vi "Write Data.vi"(8 "error in (no error)":errorcluster, 9 "Publication Time":timestamp, 10 "Value":variant, 11 "TerminalReference in":refnum<class "NamedNumericStringsBinding.lvclass">) -> (0 "error out":errorcluster, 3 "TerminalReference out":refnum<class "NamedNumericStringsBinding.lvclass">)   [LabVIEW 2017, in "Transport.lvlib" / "NamedNumericStringsBinding.lvclass"]
doc: "<License>\nCopyright © 2017 Composed Systems, LLC | All rights reserved\nwww.composed.io\n\nAuthor: Ethan Stern <ethan.stern@composed.io>\n\nThis software is provided \"AS IS\" WITHOUT WARRANTIES, either express or implied, AND IS FOR EDUCATIONAL PURPOSES ONLY.\n</License>MVA Framework 1.0.4.16\nEthan Stern - Composed Systems\nCopyright (c) 2017, Composed Systems"
uses:
  NamedNumericStringsBinding.lvclass
  NamedNumericStringsBinding.lvclass/NamedNumericStringsBinding.ctl
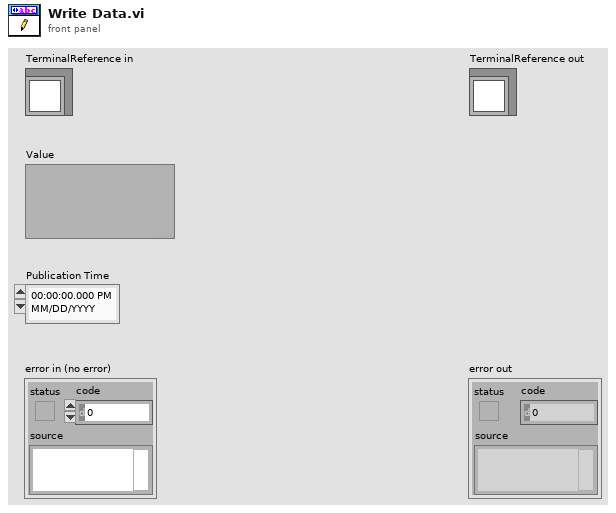
[diagram p1: front panel]
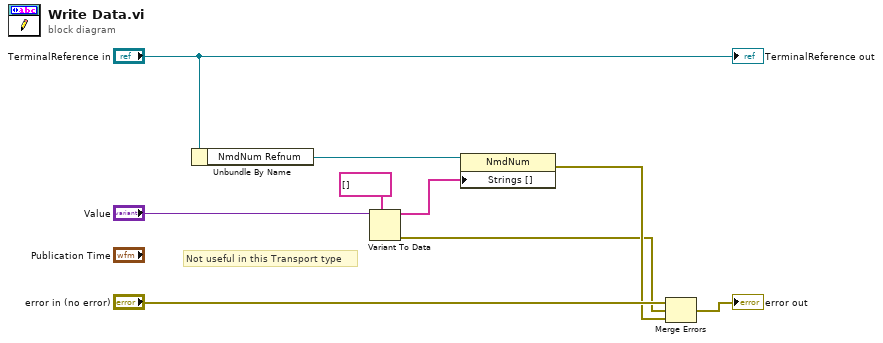
[diagram p0: block diagram]
diagram:
  # "Not useful in this Transport type"
  n1 = Unbundle By Name("TerminalReference in") -> ("NmdNum Refnum"=w7:refnum<vi>)
  n2 = Variant To Data(type=string[] [] ("Strings []"), Variant="Value") -> (data=w3:string[], error out=w1:errorcluster)  [unwired: 1 in]
  n3 = property class="NmdNum"(reference=w7, "Strings []"=w3) -> (error out=w2:errorcluster)  [unwired: 1 in, 1 out]
  n4 = Merge Errors("error in (no error)", w1, w2) -> (→"error out":errorcluster)
  "TerminalReference out" <- "TerminalReference in"
